vi "connect points.vi"(1 "waveform in":u8[](array[numeric])=[128], 2 "Coords prev":cluster{"x":i16, "y":i16}, 3 "Coords new":cluster{"x":i16, "y":i16}) -> (0 "waveform out":u8[](array[numeric]))   [LabVIEW 2009]
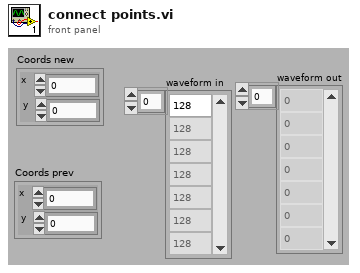
[diagram p1: front panel]
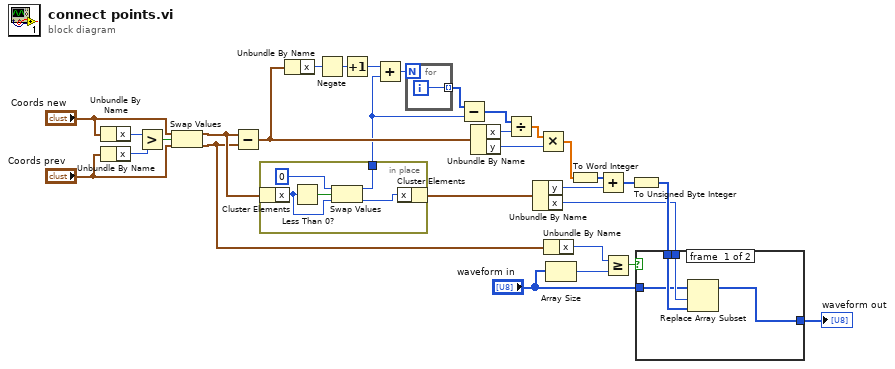
[diagram p0: block diagram]
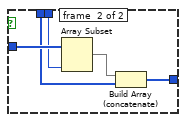
[diagram p2: hidden frame]
diagram:
  n1 = Unbundle By Name("Coords new") -> ("x"=w20:i16)
  n2 = Unbundle By Name("Coords prev") -> ("x"=w27:i16)
  n3 = Greater?(x=w20, y=w27) -> (0:w28:bool)
  n4 = Swap Values(12:"Coords new", 13:w28, 14:"Coords prev") -> (1:w9:cluster{"x":i16, "y":i16}, 3:w7:cluster{"x":i16, "y":i16})
  n5 = Subtract(x=w9, y=w7) -> (x-y=w11:cluster{"x":i16, "y":i16})
  n6 = in-place {
    in-place-border: [w34] -> w2
    n7 = in-place-cluster #1(w9) -> ("x"=w32:i16)
    n8 = Less Than 0?(x=w32) -> (x < 0?=w33:bool)
    n9 = Swap Values(12:i16 0 ("x"), 13:w33, 14:w32) -> (1:w34:i16, 3:w31:i16)
    n10 = in-place-cluster #1("x"=w31) -> (w8:cluster{"x":i16, "y":i16})
  }
  n11 = Unbundle By Name(w11) -> ("x"=w10:i16)
  n12 = Negate(x=w10) -> (-x=w6:i16)
  n13 = Increment(x=w6) -> (x+1=w5:i16)
  n14 = Add(x=w5, y=w2) -> (x+y=w4:i16)
  n15 = for {
    N: w4 -> [_]
    tunnel: [w36] -> w3 mode=indexing
    i -> [w36]
  }
  n16 = Subtract(x=w3, y=w2) -> (x-y=w1:i32[])
  n17 = Unbundle By Name(w11) -> ("x"=w24:i16, "y"=w22:i16)
  n18 = Divide(x=w1, y=w24) -> (x/y=w23:dbl[])
  n19 = Unbundle By Name(w8) -> ("y"=w16:i16, "x"=w12:i16)
  n20 = Multiply(x=w23, y=w22) -> (x*y=w17:dbl[])
  n21 = Unbundle By Name(w7) -> ("x"=w13:i16)
  n22 = Array Size(array="waveform in") -> (size(s)=w19:i32)
  n23 = To Word Integer(number=w17) -> (16bit integer=w15:i16[])
  n24 = Add(x=w15, y=w16) -> (x+y=w29:i16[])
  n25 = Greater Or Equal?(x=w13, y=w19) -> (x >= y?=w18:bool)
  n26 = To Unsigned Byte Integer(number=w29) -> (unsigned 8bit integer=w14:u8[])
  n27 = case shown="False" w18 {
    tunnel: [w40 w41] -> w30
    tunnel: w12 -> [w39 w44]
    tunnel: w14 -> [w38 w42]
    tunnel: "waveform in" -> [w37 w45]
    frame #0 {
      n28 = Replace Array Subset(array=w37, new element=w38, index=w39) -> (w40:u8[])
    }
    frame #1 {
      n29 = Array Subset(array=w45, length=w44) -> (w43:u8[])  [unwired: 1 in]
      n30 = Build Array (concatenate)(w43, w42) -> (w41:u8[])
    }
  }
  "waveform out" <- w30
